vi "senserNameToFieldIdx.vi"(8 "error in (no error)":errorcluster, 10 "Sensor Name":string, 11 "Path":path=path "/home/ttsai/Documents/stash/ts_tcs_ofc/configData/lsst/sensorNameToFieldIdx.txt") -> (0 "error out":errorcluster, 2 "Idx of Field":i32)   [LabVIEW 2016]
doc: "Transfer the abbreviate sensor name (e.g. R22_S11) to the index of optical field."
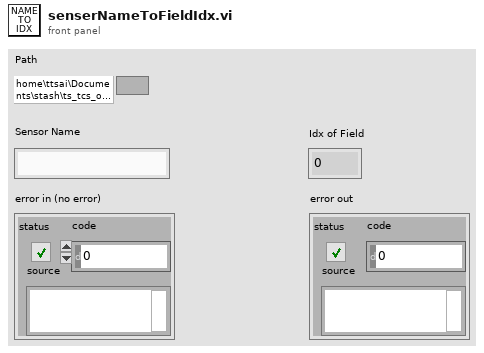
[diagram p1: front panel]
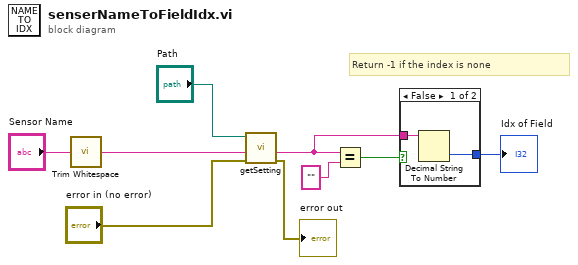
[diagram p0: block diagram]
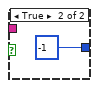
[diagram p2: hidden frame]
diagram:
  # "Return -1 if the index is none"
  n1 = call <vilib>:"Trim Whitespace.vi"("string"="Sensor Name") -> ("trimmed string"=w5:string)  [unwired: 1 in]
  n2 = call "getSetting.vi"("error in"="error in (no error)", "Parameter"=w5, "Path"="Path") -> ("error out"=→"error out":errorcluster, "Value"=w2:string)  [unwired: 7 in]
  n3 = Equal?(x=w2, y="") -> (x = y?=w3:bool)
  n4 = case shown="False" w3 {
    tunnel: w2 -> [w11 _]
    tunnel: [w10 -1] -> w1
    frame False {
      n5 = Decimal String To Number(string=w11) -> (number=w10:i32)  [unwired: 2 in, 1 out]
    }
    frame True {
    }
  }
  "Idx of Field" <- w1
